vi "UTIL_GetCalCoef.vi"(10 "Cal Table":T1={"LSe"=0.0, "LKe"=8.2, "LMe"=8.2, "LKf"=2.4, "LMf"=2.4, "LSf"=8.5}) -> (3 "Cal Coef out":T2={"M"=8.2, "B"=0.0, "Mc"=0.0, "LKe"=0.0, "LMe"=0.0})   [LabVIEW 2024]
uses:
  Control Definitions/Def CalCoef.ctl
  Control Definitions/Def CalTable.ctl
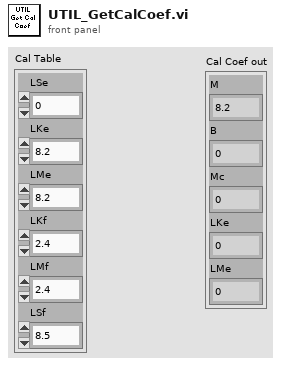
[diagram p1: front panel]
types:
  T1 = typedef "Def CalTable.ctl" = cluster{"LSe":dbl, "LKe":dbl, "LMe":dbl, "LKf":dbl, "LMf":dbl, "LSf":dbl}
  T2 = typedef "Def CalCoef.ctl" = cluster{"M":dbl, "B":dbl, "Mc":dbl, "LKe":dbl, "LMe":dbl}
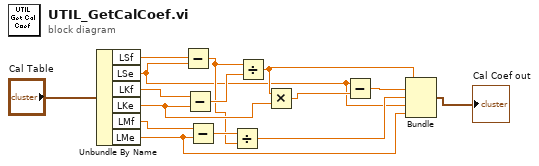
[diagram p0: block diagram]
diagram:
  n1 = Unbundle By Name("Cal Table") -> ("LSf"=w2:dbl, "LSe"=w1:dbl, "LKf"=w4:dbl, "LKe"=w13:dbl, "LMf"=w5:dbl, "LMe"=w12:dbl)
  n2 = Subtract(x=w2, y=w1) -> (x-y=w3:dbl)
  n3 = Subtract(x=w4, y=w13) -> (x-y=w7:dbl)
  n4 = Subtract(x=w5, y=w12) -> (x-y=w6:dbl)
  n5 = Divide(x=w6, y=w3) -> (x/y=w10:dbl)
  n6 = Divide(x=w3, y=w7) -> (x/y=w14:dbl)
  n7 = Multiply(x=w14, y=w13) -> (x*y=w8:dbl)
  n8 = Subtract(x=w1, y=w8) -> (x-y=w9:dbl)
  n9 = Bundle(w14, w9, w10, "LSe"=w1, "LMe"=w12) -> (→"Cal Coef out":cluster{dbl, dbl, dbl, "LSe":dbl, "LMe":dbl})  [unwired: 1 in]
